vi "Coerce with Cluster.vi"(1 "value in":dbl, 4 "output range":cluster{"high":dbl, "low":dbl}) -> (8 "coerced value":dbl, 9 "In Range?":bool)   [LabVIEW 2020]
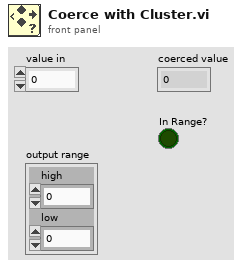
[diagram p1: front panel]
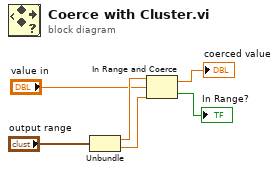
[diagram p0: block diagram]
diagram:
  n1 = Unbundle("output range") -> ("high"=w4:dbl, "low"=w5:dbl)
  n2 = In Range and Coerce(upper limit=w4, x="value in", lower limit=w5) -> (coerced(x)=→"coerced value":dbl, In Range?=→"In Range?":bool)
